vi "List Folder Files.vi"(8 "error in (no error)":errorcluster, 9 "Pattern":string="*.tdms", 10 "Folder Path":path, 11 "Batch Processor in":refnum<class "Batch Processor.lvclass">) -> (0 "error out":errorcluster, 3 "Batch Processor out":refnum<class "Batch Processor.lvclass">)   [LabVIEW 2016, in "Batch Processor.lvclass"]
uses:
  Batch Processor.lvclass
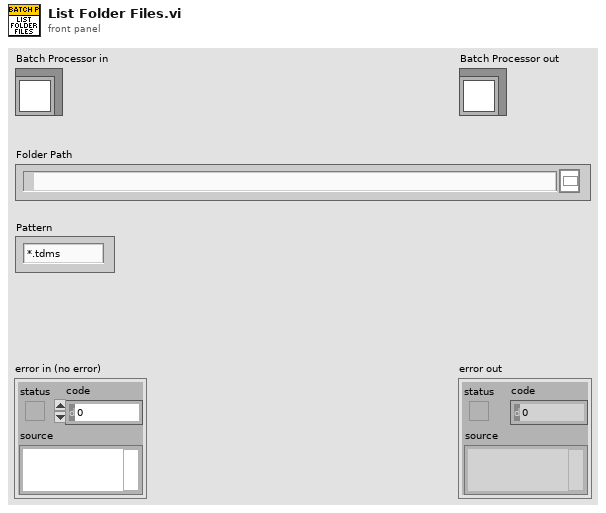
[diagram p1: front panel]
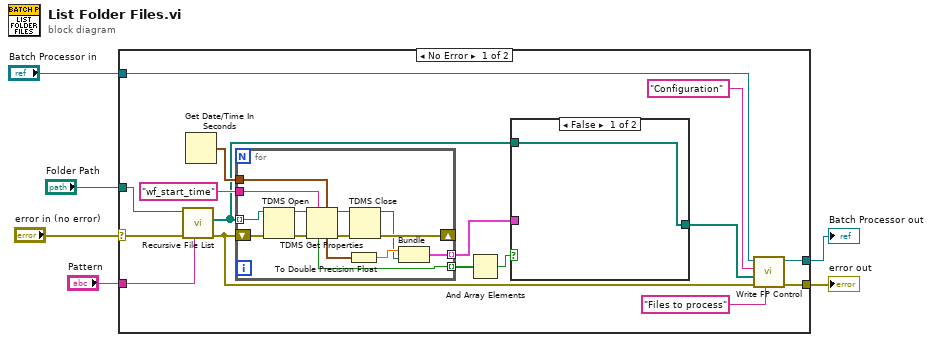
[diagram p0: block diagram]
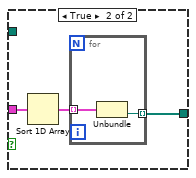
[diagram p2: hidden frame]
diagram:
  n1 = case shown="No Error" "error in (no error)" {
    selector: "error in (no error)" -> [w16 w44]
    tunnel: [w15 w44] -> w5
    tunnel: [w19 w43] -> w3
    tunnel: "Batch Processor in" -> [w22 w43]
    tunnel: "Folder Path" -> [w21 _]
    tunnel: "Pattern" -> [w20 _]
    frame No Error {
      n2 = call <vilib>:"Recursive File List.vi"("pattern"=w20, "error in (no error)"=w16, "Folder Path"=w21) -> ("error out"=w14:errorcluster, "All Files in Dir"=w7:path[])  [unwired: 4 in, 3 out]
      n3 = Get Date/Time In Seconds() -> (seconds since 1Jan1904=w12:timestamp)
      n4 = for {
        tunnel: w7 -> [w42] mode=indexing
        tunnel: "wf_start_time" -> [w38]
        tunnel: w12 -> [w37]
        shift-right: [w34] -> _
        shift-left: w14 -> [w41]
        tunnel: [w33] -> w11 mode=indexing
        tunnel: [w30] -> w10 mode=indexing
        n5 = TDMS Open(8:w41, 11:w42) -> (0:w40:errorcluster, 3:w39:refnum<k34>)  [unwired: 5 in]
        n6 = TDMS Get Properties(5:w37, 7:w38, 8:w40, 11:w39) -> (0:w36:errorcluster, 3:w35:refnum<k34>, 4:w32:timestamp, 6:w33:bool)  [unwired: 2 in, 2 out]
        n7 = To Double Precision Float(number=w32) -> (double precision float=w31:dbl)
        n8 = TDMS Close(8:w36, 11:w35) -> (0:w34:errorcluster, 3:w29:path)
        n9 = Bundle(w31, "file path out"=w29) -> (w30:cluster{dbl, "file path out":path})  [unwired: 1 in]
      }
      n10 = And Array Elements(Boolean array=w11) -> (logical AND=w9:bool)
      n11 = case shown="False" w9 {
        tunnel: w10 -> [_ w26]
        tunnel: [w23 w24] -> w8
        tunnel: w7 -> [w23 _]
        frame False {
        }
        frame True {
          n12 = Sort 1D Array(array=w26) -> (sorted array=w25:cluster{dbl, "file path out":path}[])
          n13 = for {
            tunnel: w25 -> [w28] mode=indexing
            tunnel: [w27] -> w24 mode=indexing
            n14 = Unbundle(w28) -> ("file path out"=w27:path)  [unwired: 1 out]
          }
        }
      }
      n15 = call-dynamic "Write FP Control.vi"("Field name"="Files to process", "error in (no error)"=w14, "Control Value"=w8, "Control Name"="Configuration", "Measure Object in"=w22) -> ("error out"=w15:errorcluster, "Measure Object out"=w19:refnum<class "Batch Processor.lvclass">)  [unwired: 5 in]
    }
    frame Error {
    }
  }
  "error out" <- w5
  "Batch Processor out" <- w3
